vi "HP81110A Output Set.vi"(6 "notoutput2":bool caption="Not-Output 2", 7 "output1":bool caption="Output 1", 8 "error in (no error)":errorcluster, 9 "output2":bool caption="Output 2", 10 "notoutput1":bool caption="Not-Output 1", 11 "VISA session":refnum<visa-resource-name>) -> (0 "error out":errorcluster, 3 "dup VISA session":refnum<visa-resource-name>)   [LabVIEW 2009]
doc: "This VI switches the four outputs on or off."
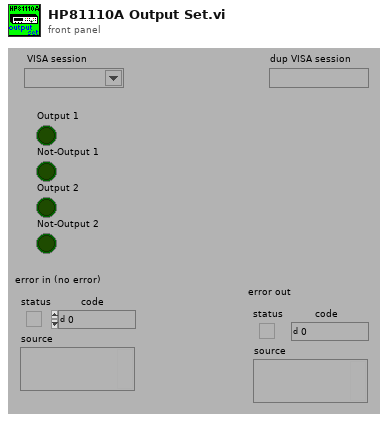
[diagram p1: front panel]
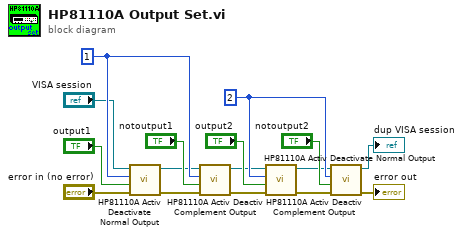
[diagram p0: block diagram]
diagram:
  w15 = 2
  w16 = 1
  n1 = call "HP81110A Activ Deactivate Normal Output.vi"("error in (no error)"="error in (no error)", "Normal State (F:Off)"="output1", "Channel (1:Channel 1)"=w16, "VISA session"="VISA session") -> ("error out"=w10:errorcluster, "dup VISA session"=w5:refnum<visa-resource-name>)  [unwired: 6 out]
  n2 = call "HP81110A Activ Deactiv Complement Output.vi"("error in (no error)"=w10, "Complement State (F:Off)"="notoutput1", "Channel (1:Channel 1)"=w16, "VISA session"=w5) -> ("error out"=w9:errorcluster, "dup VISA session"=w6:refnum<visa-resource-name>)  [unwired: 6 out]
  n3 = call "HP81110A Activ Deactivate Normal Output.vi"("error in (no error)"=w9, "Normal State (F:Off)"="output2", "Channel (1:Channel 1)"=w15, "VISA session"=w6) -> ("error out"=w8:errorcluster, "dup VISA session"=w7:refnum<visa-resource-name>)  [unwired: 6 out]
  n4 = call "HP81110A Activ Deactiv Complement Output.vi"("error in (no error)"=w8, "Complement State (F:Off)"="notoutput2", "Channel (1:Channel 1)"=w15, "VISA session"=w7) -> ("error out"=→"error out":errorcluster, "dup VISA session"=→"dup VISA session":refnum<visa-resource-name>)  [unwired: 6 out]
